vi "CardID.vi"(11 "array in":u8[](array[numeric])) -> (1 "Card ID":string, 3 "Site ID":string)   [LabVIEW 2011]
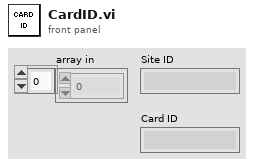
[diagram p1: front panel]
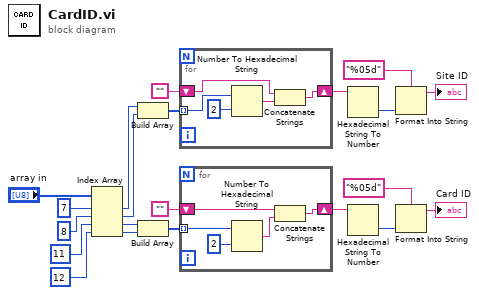
[diagram p0: block diagram]
diagram:
  n1 = Index Array(array="array in", index #1=7 ("index"), index #2=8 ("index"), index #3=11 ("index"), index #4=12 ("index")) -> (element #1=w19:u8, element #2=w18:u8, element #3=w9:u8, element #4=w8:u8)
  n2 = Build Array(w19, w18) -> (w17:u8[])
  n3 = Build Array(w9, w8) -> (w7:u8[])
  n4 = for {
    tunnel: w17 -> [w25] mode=indexing
    shift-right: [w22] -> w15
    shift-left: "" -> [w23]
    n5 = Number To Hexadecimal String(1:i16 2 ("width (-)"), 2:w25) -> (0:w24:string)
    n6 = Concatenate Strings(w23, w24) -> (w22:string)
  }
  n7 = for {
    tunnel: w7 -> [w30] mode=indexing
    shift-right: [w27] -> w3
    shift-left: "" -> [w28]
    n8 = Number To Hexadecimal String(1:i16 2 ("width (-)"), 2:w30) -> (0:w29:string)
    n9 = Concatenate Strings(w28, w29) -> (w27:string)
  }
  n10 = Hexadecimal String To Number(string=w15) -> (number=w14:u32)  [unwired: 2 in, 1 out]
  n11 = Hexadecimal String To Number(string=w3) -> (number=w4:u32)  [unwired: 2 in, 1 out]
  n12 = Format Into String(format string="%05d", w14) -> (resulting string=→"Site ID":string)  [unwired: 2 in, 1 out]
  n13 = Format Into String(format string="%05d", w4) -> (resulting string=→"Card ID":string)  [unwired: 2 in, 1 out]
